vi "Expert_ResetAllDevices.vi"(7 "Error IN Toolkit":i32, 11 "Error IN LabVIEW":errorcluster) -> (8 "Error OUT Toolkit":i32, 15 "Error OUT LabVIEW":errorcluster)   [LabVIEW 2018]
doc: "It resets all GPU devices. In case this VI is not initial, an error integer must be passed from a VI that uses the same DLL to avoid errors."
uses:
  dll/LibreriaAutis_3.dll
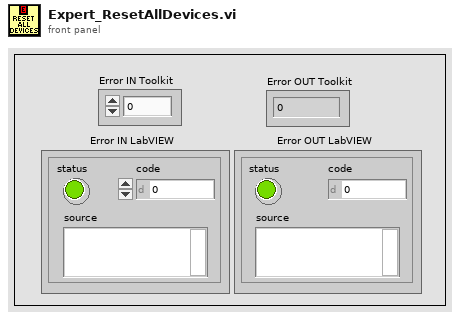
[diagram p1: front panel]
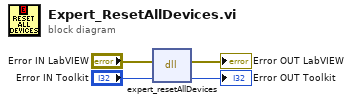
[diagram p0: block diagram]
diagram:
  n1 = dll-call lib="C:/Users/AUTIS/Desktop/LibreriaAUTIS/LabVIEW/dll/LibreriaAutis_3.dll" fn="expert_resetAllDevices"(error in="Error IN LabVIEW", "error"="Error IN Toolkit") -> (error out=→"Error OUT LabVIEW":errorcluster, "error"=→"Error OUT Toolkit":i32)  [unwired: 3 in, 1 out]
